vi "3DDataTrain.vi"(7 "Index":cluster{"X":i32, "Y":i32, "Z":i32}, 8 "error in":errorcluster, 10 "Y":dbl[](array[numeric]), 11 "X":dbl[][](array[numeric])) -> (0 "error out":errorcluster, 3 "3DArray":cluster{"X":dbl[], "Y":dbl[], "Z":dbl[]}[](array[cluster]))   [LabVIEW 2020]
doc: "Rearrange the Train data"
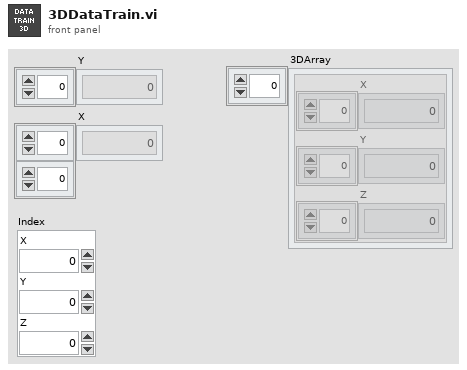
[diagram p1: front panel]
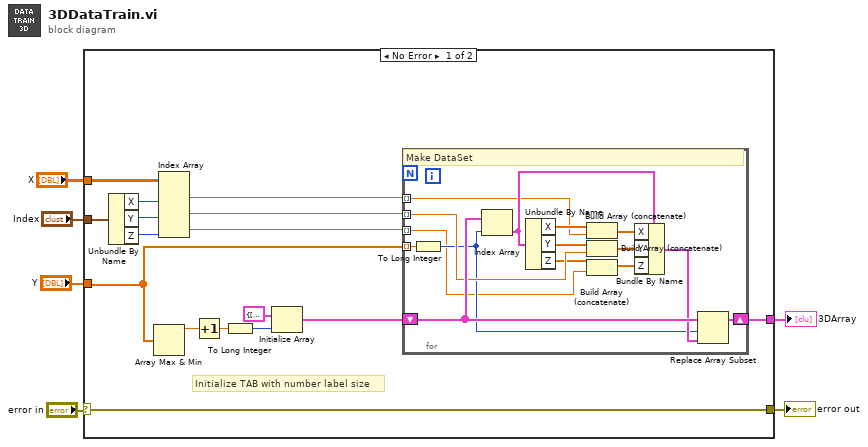
[diagram p0: block diagram]
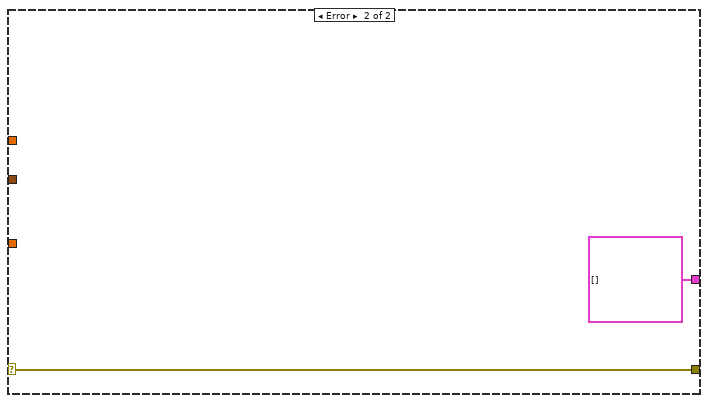
[diagram p2: hidden frame]
diagram:
  n1 = case shown="No Error" "error in" {
    selector: "error in" -> [w22 w39]
    tunnel: "X" -> [w10 _]
    tunnel: "Y" -> [w9 _]
    tunnel: [w22 w39] -> w2
    tunnel: "Index" -> [w8 _]
    tunnel: [w7 cluster{"X":dbl[], "Y":dbl[], "Z":dbl[]}[] []] -> w1
    frame No Error {
      # "Initialize TAB with number label size"
      n2 = Unbundle By Name(w8) -> ("X"=w21:i32, "Y"=w20:i32, "Z"=w19:i32)
      n3 = Array Max & Min(array=w9) -> (max value=w16:dbl)  [unwired: 3 out]
      n4 = Index Array(array=w10, index (col) #1=w21, index (col) #2=w20, index (col) #3=w19) -> (element #1=w13:dbl[], element #2=w12:dbl[], element #3=w11:dbl[])  [unwired: 3 in]
      n5 = Increment(x=w16) -> (x+1=w18:dbl)
      n6 = To Long Integer(number=w18) -> (32bit integer=w14:i32)
      n7 = Initialize Array(cluster{"X":dbl[], "Y":dbl[], "Z":dbl[]} {"X"=[], "Y"=[], "Z"=[]} ("Cluster"), w14) -> (w17:cluster{"X":dbl[], "Y":dbl[], "Z":dbl[]}[])
      n8 = for {
        tunnel: w12 -> [w29] mode=indexing
        tunnel: w13 -> [w27] mode=indexing
        tunnel: w9 -> [w31] mode=indexing
        shift-right: [w33] -> w7
        shift-left: w17 -> [w34]
        tunnel: w11 -> [w24] mode=indexing
        # "Make DataSet"
        n9 = To Long Integer(number=w31) -> (32bit integer=w26:i32)
        n10 = Index Array(array=w34, index=w26) -> (element=w37:cluster{"X":dbl[], "Y":dbl[], "Z":dbl[]})
        n11 = Unbundle By Name(w37) -> ("X"=w28:dbl[], "Y"=w30:dbl[], "Z"=w25:dbl[])
        n12 = Build Array (concatenate)(w28, w27) -> (w36:dbl[])
        n13 = Build Array (concatenate)(w30, w29) -> (w35:dbl[])
        n14 = Build Array (concatenate)(w25, w24) -> (w23:dbl[])
        n15 = Bundle By Name(cluster=w37, "X"=w36, "Y"=w35, "Z"=w23) -> (w32:cluster{"X":dbl[], "Y":dbl[], "Z":dbl[]})
        n16 = Replace Array Subset(array=w34, new element=w32, index=w26) -> (w33:cluster{"X":dbl[], "Y":dbl[], "Z":dbl[]}[])
      }
    }
    frame Error {
    }
  }
  "error out" <- w2
  "3DArray" <- w1
